vi "Waveform, Calculate RMS Jitter.vi"(0 "error in":errorcluster, 3 "waveform":waveform(dbl)={"t0"=timestamp(3473168073.631 s since 1904-01-01), "dt"=1e-08, "Y"=[], "attributes"=variant("Average Size"=variant(dbl 15.0), "NSamp"=variant(dbl 400000.0), "Resistance (ohms)"=variant(dbl 500.0), "Samp Freq (MHz)"=variant(dbl 100.0), "dt (us)"=variant(dbl 0.01))}, 4 "transition index":dbl[](array[numeric])) -> (7 "error out":errorcluster, 8 "Frequency (Hz)":dbl=nan format="%.3f", 9 "Period Jitter (us rms)":dbl=nan format="%.3f", 10 "waveform dup":waveform(dbl)={"t0"=timestamp(-9593190233.15 s since 1904-01-01), "dt"=nan, "Y"=[], "attributes"=variant("Average Size"=variant(dbl 15.0), "NSamp"=variant(dbl 113636.0), "Resistance (ohms)"=variant(dbl 10000.0), "Samp Freq (MHz)"=variant(dbl 0.5), "dt (us)"=variant(dbl 2.0))})   [LabVIEW 2010]
doc: "This function calculates Frequency (Hz) and Period Jitter (us rms) using standard deviation per the IEEE standard.\n\nNo instrument jitter correction is calculated, since the instrument jitter should be insignificant compared to the measured waveform.\n\nThe National Instruments PXI-5122 Digitizer Trigger Jitter is less than 80 ps rms, clock jitter is 2 ps rms."
uses:
  <vilib>/Analysis/NI_AALBase.lvlib
panel:
  out "periods":dbl[](array[numeric])
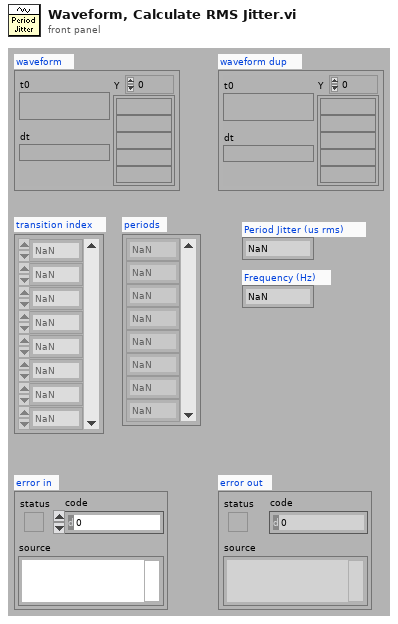
[diagram p1: front panel]
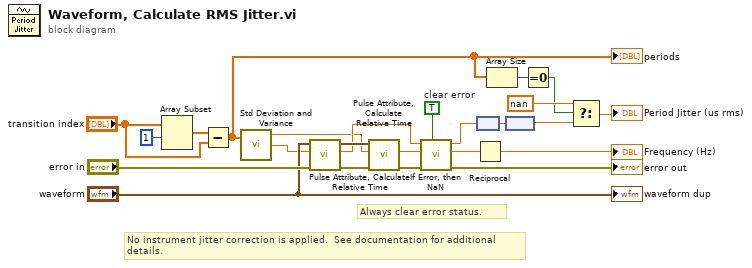
[diagram p0: block diagram]
diagram:
  w23 = TRUE  # clear error
  # "No instrument jitter correction is applied.  See documentation for additional details."
  # "Always clear error status."
  n1 = Array Subset(array="transition index", index=1) -> (w19:dbl[])  [unwired: 1 in]
  n2 = Subtract(x=w19, y="transition index") -> (x-y=w2:dbl[])
  "periods" <- w2
  n3 = call <vilib>:"Std Deviation and Variance.vi"("X"=w2) -> ("mean"=w10:dbl, "standard deviation"=w11:dbl)  [unwired: 1 in, 1 out]
  n4 = call "Pulse Attribute, Calculate Relative Time.vi"("error in"="error in", "index"=w11, "waveform"="waveform") -> ("error out"=w16:errorcluster, "relative time (s)"=w12:dbl, "waveform dup"=w15:waveform(dbl))  [unwired: 4 in]
  n5 = call "Pulse Attribute, Calculate Relative Time.vi"("error in"=w16, "index"=w10, "waveform"=w15) -> ("error out"=w21:errorcluster, "relative time (s)"=w13:dbl)  [unwired: 4 in, 1 out]
  n6 = call "If Error, then NaN.vi"("clear error (F)"=w23, "error in (T)"=w21, "value2"=w13, "value1"=w12) -> ("error out"=→"error out":errorcluster, "value out2"=w8:dbl, "value out1"=w9:dbl)  [unwired: 2 in, 1 out]
  n7 = Reciprocal(x=w8) -> (1/x=→"Frequency (Hz)":dbl)
  n8 = node(w9) -> (w22:dbl[unit])
  n9 = Array Size(array=w2) -> (size(s)=w3:i32)
  n10 = node(w22) -> (w6:dbl)
  n11 = Equal To 0?(x=w3) -> (x = 0?=w1:bool)
  n12 = Select(t=nan, s=w1, f=w6) -> (s? t:f=→"Period Jitter (us rms)":dbl)
  "waveform dup" <- "waveform"
